vi "BRig_RT__Case_Idle__State_RewardCalibration_pre.vi"(0 "input_dataMTrig":u16[](array[numeric]), 2 "Solenoid_Tcycle_L":u16=300, 3 "Solenoid_Tcycle_R":u16=300, 5 "RewCalib_Ncycle__L":u16=100, 6 "RewCalib_Ncycle__R":u16=100, 10 "RewCalib_Trig_L":bool caption="Calibrate_L", 12 "RewCalib_Trig_R":bool caption="Calibrate_R") -> (20 "output_dataMTrig":u16[](array[numeric]))   [LabVIEW 2014]
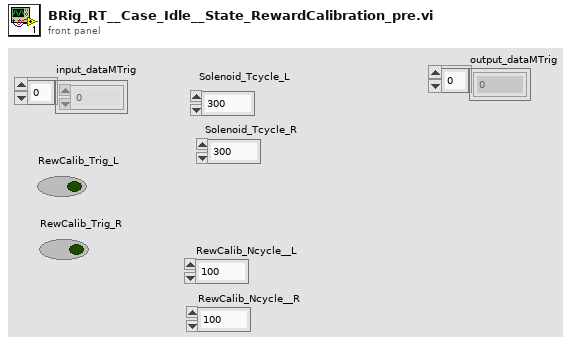
[diagram p1: front panel]
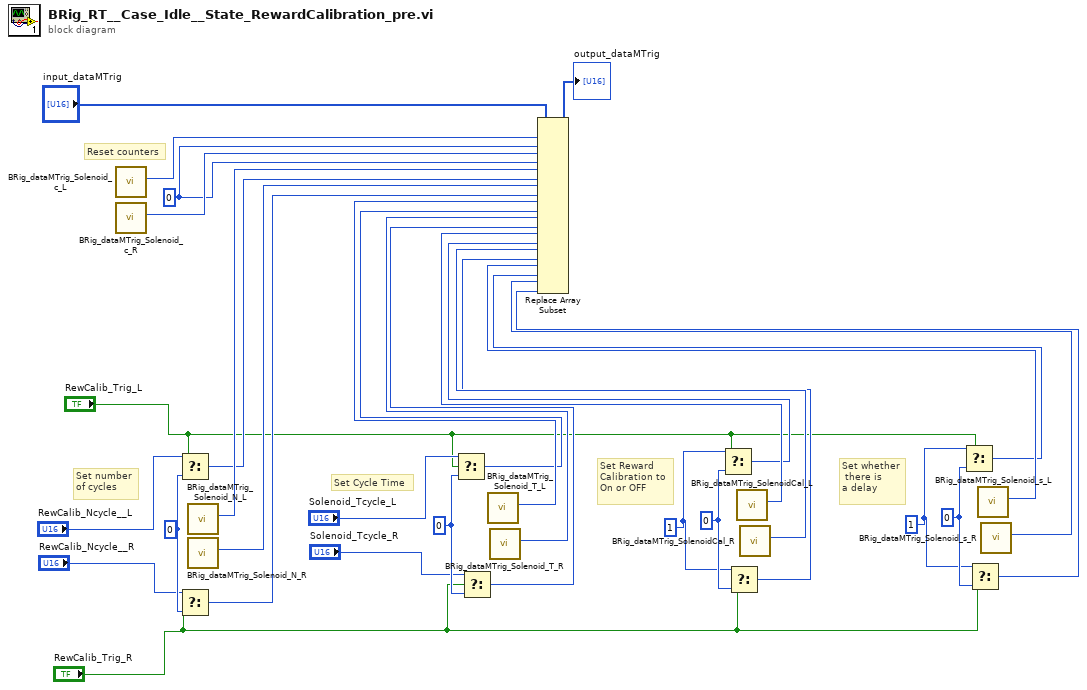
[diagram p0: block diagram]
diagram:
  w7 = 1 ("t")
  w8 = 0 ("f")
  w19 = 1 ("t")
  w20 = 0 ("f")
  w25 = 0 ("f")
  w30 = 0 ("f")
  w31 = u32 0 ("new element/subarray")
  # "Set whether\n there is\na delay"
  # "Set Reward\nCalibration to\nOn or OFF"
  # "Set Cycle Time"
  # "Set number\nof cycles"
  # "Reset counters"
  n1 = call "BRig_dataMTrig_Solenoid_c_L.vi"() -> ("output_Solenoid_c_L"=w33:i32)  [unwired: 11 in]
  n2 = call "BRig_dataMTrig_Solenoid_c_R.vi"() -> ("output_Solenoid_c_R"=w32:i32)  [unwired: 11 in]
  n3 = Select(t="RewCalib_Ncycle__L", s="RewCalib_Trig_L", f=w30) -> (s? t:f=w27:i32)
  n4 = Select(t="RewCalib_Ncycle__R", s="RewCalib_Trig_R", f=w30) -> (s? t:f=w26:i32)
  n5 = call "BRig_dataMTrig_Solenoid_N_L.vi"() -> ("output_Solenoid_N_L"=w29:i32)  [unwired: 11 in]
  n6 = call "BRig_dataMTrig_Solenoid_N_R.vi"() -> ("output_Solenoid_N_R"=w28:i32)  [unwired: 11 in]
  n7 = Select(t="Solenoid_Tcycle_L", s="RewCalib_Trig_L", f=w25) -> (s? t:f=w23:i32)
  n8 = Select(t="Solenoid_Tcycle_R", s="RewCalib_Trig_R", f=w25) -> (s? t:f=w21:i32)
  n9 = call "BRig_dataMTrig_Solenoid_T_L.vi"() -> ("output_Solenoid_T_L"=w24:i32)  [unwired: 11 in]
  n10 = call "BRig_dataMTrig_Solenoid_T_R.vi"() -> ("output_Solenoid_T_R"=w22:i32)  [unwired: 11 in]
  n11 = Select(t=w19, s="RewCalib_Trig_L", f=w20) -> (s? t:f=w17:i32)
  n12 = Select(t=w19, s="RewCalib_Trig_R", f=w20) -> (s? t:f=w15:i32)
  n13 = call "BRig_dataMTrig_SolenoidCal_L.vi"() -> ("output_SolenoidCal_L"=w18:i32)  [unwired: 11 in]
  n14 = call "BRig_dataMTrig_SolenoidCal_R.vi"() -> ("output_SolenoidCal_R"=w16:i32)  [unwired: 11 in]
  n15 = Select(t=w7, s="RewCalib_Trig_L", f=w8) -> (s? t:f=w2:i32)
  n16 = Select(t=w7, s="RewCalib_Trig_R", f=w8) -> (s? t:f=w1:i32)
  n17 = call "BRig_dataMTrig_Solenoid_s_L.vi"() -> ("output_Solenoid_s_L"=w4:i32)  [unwired: 11 in]
  n18 = call "BRig_dataMTrig_Solenoid_s_R.vi"() -> ("output_Solenoid_s_R"=w3:i32)  [unwired: 11 in]
  n19 = Replace Array Subset(array="input_dataMTrig", new element #1=w31, index #1=w33, new element #2=w31, index #2=w32, new element #3=w27, index #3=w29, new element #4=w26, index #4=w28, new element #5=w23, index #5=w24, new element #6=w21, index #6=w22, new element #7=w17, index #7=w18, new element #8=w15, index #8=w16, new element #9=w2, index #9=w4, new element #10=w1, index #10=w3) -> (→"output_dataMTrig":u16[])
